vi "Read Boolean Text.vi"(8 "error in":errorcluster, 11 "Boolean Reference in":refnum<vi>) -> (0 "error out":errorcluster, 1 "Interpret As Unicode":bool, 2 "Value":string[](array[string]), 3 "Boolean Reference out":refnum<vi>)   [LabVIEW 2020, in "G-Unicode.lvlib"]
uses:
  G-Unicode.lvlib
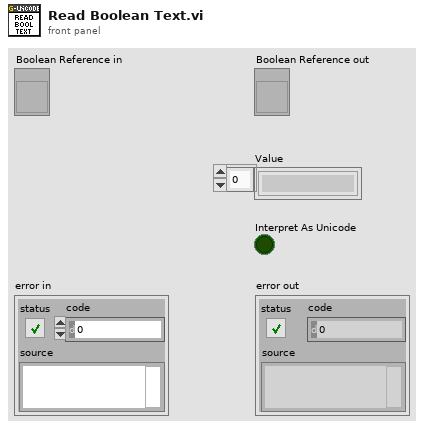
[diagram p1: front panel]
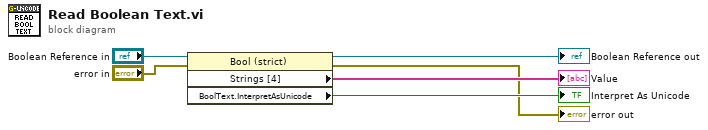
[diagram p0: block diagram]
diagram:
  n1 = property class="Bool (strict)"(reference="Boolean Reference in", error in="error in") -> (reference out=→"Boolean Reference out":refnum<vi>, error out=→"error out":errorcluster, "Strings [4]"=→"Value":string[], "BoolText.InterpretAsUnicode"=→"Interpret As Unicode":bool)
